vi "MoveGrid.vi"(7 "type":u16(ring)=1 items=["Line", "Grid", "Cloud"], 8 "y":sgl, 9 "x":sgl, 10 "error in (no error)":errorcluster, 11 "Application ref in":refnum<vi>) -> (2 "error out":errorcluster, 3 "Application ref out":refnum<vi>)   [LabVIEW 2021]
uses:
  <userlib>/Nanonis Prog Interface V5/Scan/Grid/LinePatternGet.vi
  <userlib>/Nanonis Prog Interface V5/Scan/Grid/LinePatternSet.vi
  <userlib>/Nanonis Prog Interface V5/Scan/Grid/CloudPatternGet.vi
  <userlib>/Nanonis Prog Interface V5/Scan/Grid/CloudPatternSet.vi
  <userlib>/Nanonis Prog Interface V5/Scan/Grid/GridPatternGet.vi
  <userlib>/Nanonis Prog Interface V5/Scan/Grid/GridPatternSet.vi
  <userlib>/Nanonis Prog Interface V5/Nanonis Prog Interface.lvlib
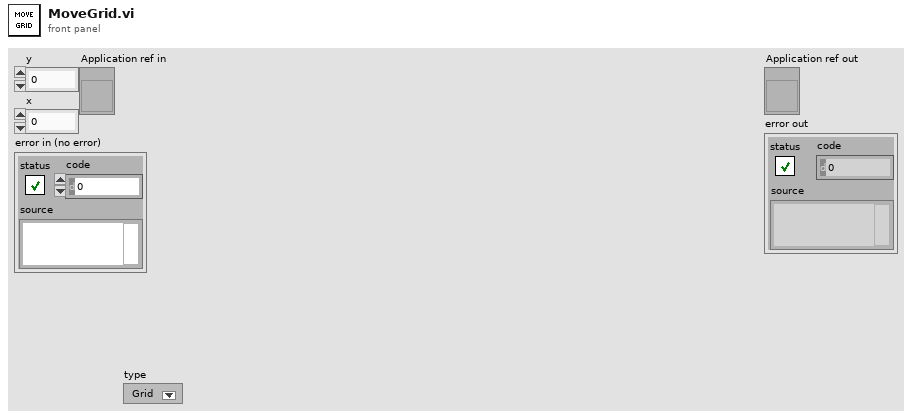
[diagram p1: front panel]
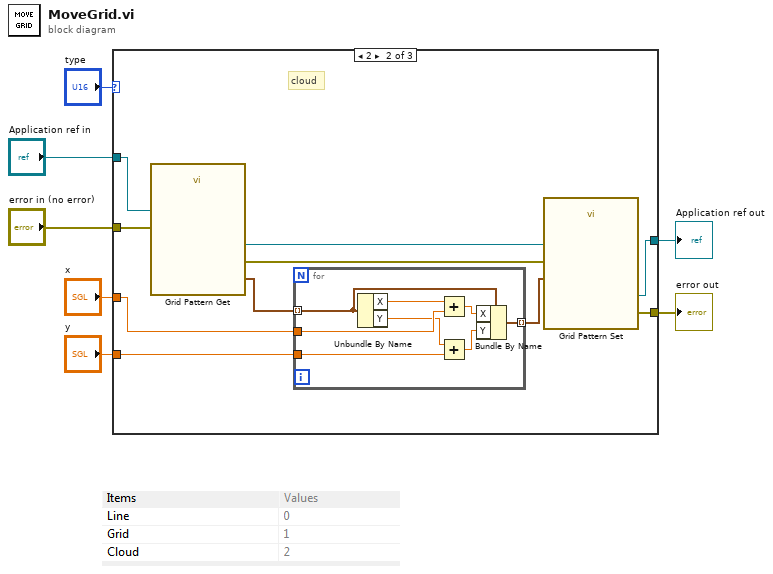
[diagram p0: block diagram]
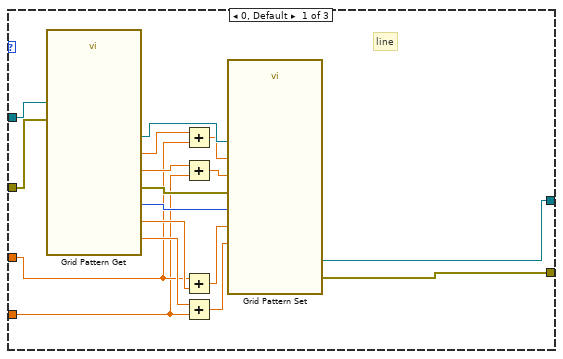
[diagram p2: hidden frame]
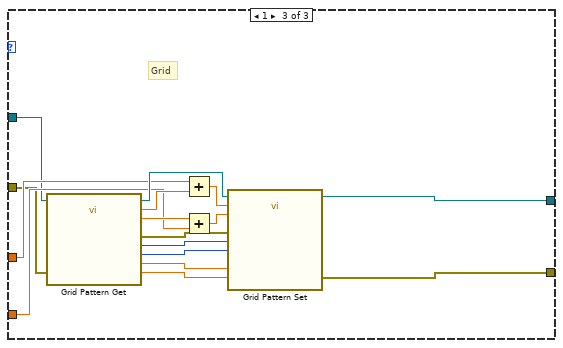
[diagram p3: hidden frame]
diagram:
  n1 = case shown="2" "type" {
    tunnel: "y" -> [w8 w25 w52]
    tunnel: "x" -> [w9 w26 w51]
    tunnel: "Application ref in" -> [w18 w32 w50]
    tunnel: [w17 w31 w49] -> w4
    tunnel: "error in (no error)" -> [w16 w30 w48]
    tunnel: [w15 w29 w47] -> w2
    frame 0, Default {
      # "line"
      n2 = call-poly <userlib>:"Grid Pattern Get.vi"("Application ref in"=w18, "error in (no error)"=w16) -> ("Points"=w14:i32, "Application ref out"=w24:refnum<vi>, "Start X1 (m)"=w22:sgl, "Start Y1 (m)"=w21:sgl, "End X2 (m)"=w13:sgl, "End Y2 (m)"=w11:sgl, "error out"=w23:errorcluster)  [unwired: 11 in]
      n3 = Add(x=w13, y=w9) -> (x+y=w12:sgl)
      n4 = Add(x=w11, y=w8) -> (x+y=w10:sgl)
      n5 = Add(x=w9, y=w22) -> (x+y=w20:sgl)
      n6 = Add(x=w21, y=w8) -> (x+y=w19:sgl)
      n7 = call-poly <userlib>:"Grid Pattern Set.vi"("Application ref in"=w24, "Start X1 (m) (NaN=no change)"=w20, "Start Y1 (m) (NaN=no change)"=w19, "End X2 (m) (NaN=no change)"=w12, "End Y2 (m) (NaN=no change)"=w10, "error in (no error)"=w23, "Points (0=no change)"=w14) -> ("Application ref out"=w17:refnum<vi>, "error out"=w15:errorcluster)  [unwired: 11 in]
    }
    frame 2 {
      # "cloud"
      n8 = call-poly <userlib>:"Grid Pattern Get.vi"("Application ref in"=w32, "error in (no error)"=w30) -> ("Application ref out"=w34:refnum<vi>, "Cloud data"=w28:cluster{"X":sgl, "Y":sgl}[], "error out"=w33:errorcluster)  [unwired: 15 in]
      n9 = for {
        tunnel: w28 -> [w42] mode=indexing
        tunnel: [w41] -> w27 mode=indexing
        tunnel: w26 -> [w38]
        tunnel: w25 -> [w35]
        n10 = Unbundle By Name(w42) -> ("X"=w40:sgl, "Y"=w37:sgl)
        n11 = Add(x=w40, y=w38) -> (x+y=w39:sgl)
        n12 = Add(x=w37, y=w35) -> (x+y=w36:sgl)
        n13 = Bundle By Name(cluster=w42, "X"=w39, "Y"=w36) -> (w41:cluster{"X":sgl, "Y":sgl})
      }
      n14 = call-poly <userlib>:"Grid Pattern Set.vi"("Application ref in"=w34, "Cloud data ( no change=default)"=w27, "error in (no error)"=w33) -> ("Application ref out"=w31:refnum<vi>, "error out"=w29:errorcluster)  [unwired: 15 in]
    }
    frame 1 {
      # "Grid"
      n15 = call-poly <userlib>:"Grid Pattern Get.vi"("Application ref in"=w50, "error in (no error)"=w48) -> ("Height (m)"=w45:sgl, "Points Y"=w43:i32, "Width (m)"=w46:sgl, "Points X"=w44:i32, "Application ref out"=w58:refnum<vi>, "Center Xc (m)"=w56:sgl, "Center Yc (m)"=w55:sgl, "error out"=w57:errorcluster)  [unwired: 9 in, 1 out]
      n16 = Add(x=w51, y=w56) -> (x+y=w54:sgl)
      n17 = Add(x=w55, y=w52) -> (x+y=w53:sgl)
      n18 = call-poly <userlib>:"Grid Pattern Set.vi"("Application ref in"=w58, "Center Xc (m) (NaN=no change)"=w54, "Center Yc (m) (NaN=no change)"=w53, "error in (no error)"=w57, "Width (m) (NaN=no change)"=w46, "Points X (0=no change)"=w44, "Height (m) (NaN=no change)"=w45, "Points Y (0=no change)"=w43) -> ("Application ref out"=w49:refnum<vi>, "error out"=w47:errorcluster)  [unwired: 10 in]
    }
  }
  "Application ref out" <- w4
  "error out" <- w2
